vi "綜合圓軌跡子VI.vi"(0 "Ring":T1, 2 "移動z":dbl, 3 "al":dbl min=0.0, 4 "I時間":i32, 5 "be":dbl min=0.0) -> (6 "Z":dbl, 7 "A":dbl, 8 "B":dbl)   [LabVIEW 2019]
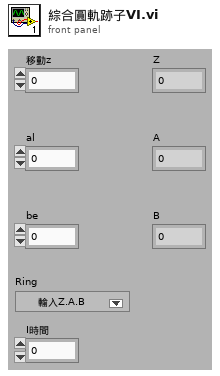
[diagram p1: front panel]
types:
  T1 = typedef "­y¸ñ.ctl" = u16
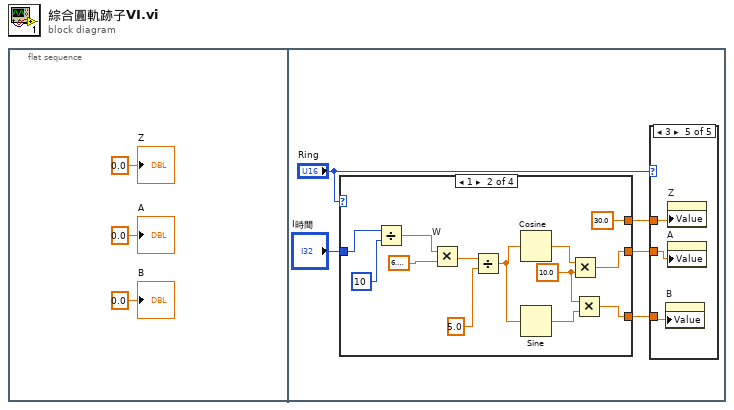
[diagram p0: block diagram]
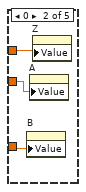
[diagram p3: hidden frame]
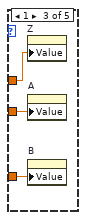
[diagram p4: hidden frame]
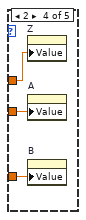
[diagram p5: hidden frame]
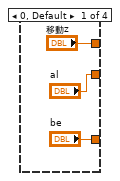
[diagram p6: hidden frame]
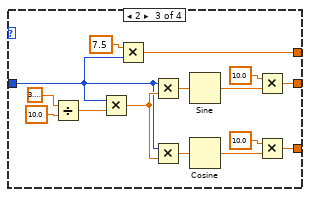
[diagram p7: hidden frame]
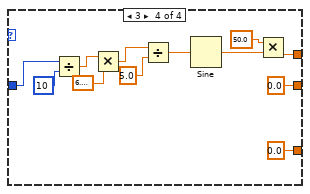
[diagram p8: hidden frame]
diagram:
  n1 = flat-sequence {
    frame #0 {
      "A" <- 0.0 ("A")
      "B" <- 0.0 ("B")
      "Z" <- 0.0 ("Z")
    }
    frame #1 {
      n2 = case shown="1" "Ring" {
        tunnel: ["移動z" 30.0 ("移動z") w39 w61] -> w4
        tunnel: ["al" w31 w38 0.0 ("al")] -> w6
        tunnel: ["be" w30 w37 0.0 ("be")] -> w7
        tunnel: "I時間" -> [_ w29 w40 w58]
        frame 0, Default {
        }
        frame 1 {
          w34 = 10.0 ("y")
          n3 = Divide(x=w29, y=10) -> (x/y=w27:dbl)
          n4 = Multiply "W"(x=w27, y=6.283185307179586) -> (x*y=w25:dbl)
          n5 = Divide(x=w25, y=5.0) -> (x/y=w26:dbl)
          n6 = Cosine(x=w26) -> (cos(x)=w32:dbl)
          n7 = Sine(x=w26) -> (sin(x)=w33:dbl)
          n8 = Multiply(x=w32, y=w34) -> (x*y=w31:dbl)
          n9 = Multiply(x=w34, y=w33) -> (x*y=w30:dbl)
        }
        frame 2 {
          n10 = Divide(x=3.141592653589793, y=10.0) -> (x/y=w48:dbl)
          n11 = Multiply(x=w40, y=w48) -> (x*y=w46:dbl)
          n12 = Multiply(x=7.5, y=w40) -> (x*y=w39:dbl)
          n13 = Multiply(x=w40, y=w46) -> (x*y=w43:dbl)
          n14 = Multiply(x=w40, y=w46) -> (x*y=w47:dbl)
          n15 = Sine(x=w43) -> (sin(x)=w45:dbl)
          n16 = Cosine(x=w47) -> (cos(x)=w44:dbl)
          n17 = Multiply(x=10.0, y=w45) -> (x*y=w38:dbl)
          n18 = Multiply(x=10.0, y=w44) -> (x*y=w37:dbl)
        }
        frame 3 {
          n19 = Divide(x=w58, y=10) -> (x/y=w57:dbl)
          n20 = Multiply(x=w57, y=6.283185307179586) -> (x*y=w55:dbl)
          n21 = Divide(x=w55, y=5.0) -> (x/y=w53:dbl)
          n22 = Sine(x=w53) -> (sin(x)=w63:dbl)
          n23 = Multiply(x=50.0, y=w63) -> (x*y=w61:dbl)
        }
      }
      n24 = case shown="3" "Ring" {
        tunnel: w4 -> [_ w11 w14 w17 w20]
        tunnel: w6 -> [_ w10 w13 w16 w19]
        tunnel: w7 -> [_ w9 w12 w15 w18]
        frame Default {
        }
        frame 0 {
          n25 = property on="B" class="DigNum (strict)"("Value"=w9) -> ()  [unwired: 2 in, 2 out]
          n26 = property on="A" class="DigNum (strict)"("Value"=w10) -> ()  [unwired: 2 in, 2 out]
          n27 = property on="Z" class="DigNum (strict)"("Value"=w11) -> ()  [unwired: 2 in, 2 out]
        }
        frame 1 {
          n28 = property on="Z" class="DigNum (strict)"("Value"=w14) -> ()  [unwired: 2 in, 2 out]
          n29 = property on="A" class="DigNum (strict)"("Value"=w13) -> ()  [unwired: 2 in, 2 out]
          n30 = property on="B" class="DigNum (strict)"("Value"=w12) -> ()  [unwired: 2 in, 2 out]
        }
        frame 2 {
          n31 = property on="Z" class="DigNum (strict)"("Value"=w17) -> ()  [unwired: 2 in, 2 out]
          n32 = property on="A" class="DigNum (strict)"("Value"=w16) -> ()  [unwired: 2 in, 2 out]
          n33 = property on="B" class="DigNum (strict)"("Value"=w15) -> ()  [unwired: 2 in, 2 out]
        }
        frame 3 {
          n34 = property on="B" class="DigNum (strict)"("Value"=w18) -> ()  [unwired: 2 in, 2 out]
          n35 = property on="Z" class="DigNum (strict)"("Value"=w20) -> ()  [unwired: 2 in, 2 out]
          n36 = property on="A" class="DigNum (strict)"("Value"=w19) -> ()  [unwired: 2 in, 2 out]
        }
      }
    }
  }
